vi "FestoCPX.Station.Laser.Shutterlock.vi"(8 "error in":errorcluster, 9 "Wait (T)":bool=TRUE, 10 "Shutterlock":bool) -> (0 "error out":errorcluster)   [LabVIEW 2015]
uses:
  FestoCPX.DO.Signal.ctl
  tools/EventLog/EventLog.EventSource.ctl
  tools/Translator/Translator.Message.ctl
  V7310/LowLevel/V7310.LaserStatus.ctl
  V7310/V7310.Data.Status.State.ctl
  FestoCPX.DO.Data.State.Set.vi
  V7310/LowLevel/V7310.Global.vi
  tools/EventLog/EventLog.CreateError(single).vi
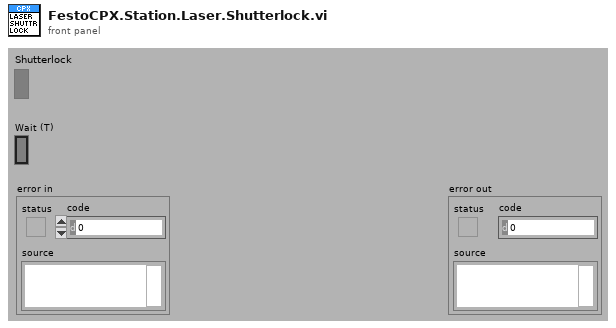
[diagram p1: front panel]
types:
  T1 = typedef "FestoCPX.DO.Signal.ctl" = enum16{"Safety Reset", "Air Main Valve", "Door Lock", "Button LED Start", "Button LED Stop", "Button LED Control", "Traffic LED Red", "Traffic LED Orange", "Traffic LED Green", "Horn", "Laser Interlock", "Laser Shutterlock", "Laser Fume Extractor", "Product Suction Gripper Slot 1 A", "Product Suction Gripper Slot 1 B", "Product Suction Gripper Slot 2 A", "Product Suction Gripper Slot 2 B", "Product Suction Gripper Slot 3 A", "Product Suction Gripper Slot 3 B", "Product Suction Gripper Slot 4 A", "Product Suction Gripper Slot 4 B", "Product Suction Gripper Final A", "Product Suction Gripper Final B", "Lamp", "Q1 Product Move Work", "Q1 Product Move Home", "Q2 Table Turn Work", "Q2 Table Turn Home", "Q3 Product Lift A", "Q3 Product Lift B", "Q4 Product Arm OK", "Q4 Product Arm NOK", "Q5 Product Arm Work"}
  T2 = typedef "Translator.Message.ctl" = enum16{"-", "Event confirmed", "Log out", "Log in", "Shutdown", "Cancel", "Start", "Begin time", "End time", "Duration", "Service Mode", "Ignore Results", "On", "Off", "OK", "NOK", "NOK %s", "Home", "Work", "Close", "Open", "In progress...", "Missing", "Empty", "Hardware failure", "Initial", "Error %d >> %s", "Error %d >> %s >> %s", "Msg %d >> %s", "Laser cmd error %s %d", "Laser cmd failed %s", "Laser cmd warning %s", "Laser disconnected", "Laser status %s", "Laser already started", "Laser job unkonwn %s", "Laser job missing %s", "Laser job select failure %s", "Laser marking timeout", "Laser marking aborted", "Unable to reset Laser Interlock (%s)", "Unable to trigger Laser. Laser not ready (%s)", "Starting %s", "Quitting %s", "Configured", "Initializing", "Quitting", "Loading", "Running", "Stopped", "Summary", "Laser", "Do you want to continue?", "Press confirm button", "Station is not based. Do you want to exit?", "Station requires changeover. Do you want to run the test?", "Test options are not set as default. Do you want to continue?", "Product not detected. Do you want to continue?", "Product scan failed. Do you want to continue?", "Calibration", "Log out?", "System", "All", "IDLE", "Translating...%s", "Not found", "Alarm %s", "Run", "Skip", "Abort", "Repeat", "Please wait...", "Database disconnected", "Database disconnected - changeover disabled!", "Login to database successful", "Login to database failed: %d; %s", "Unable to check the product status of reference %d - database disconnected", "Unable to set the product status of reference %d - database disconnected", "Variant file backup %s", "Read steps (%s)", "Result", "Station armed!", "Station requires changeover!", "Select reference number...", "EMERGENCY BUTTON - press Control button", "EMERGENCY DOOR - press Control button", "Resetting Emergency...", "Unable to reset safety circuit - Emergency Button pressed", "Unable to reset safety circuit - Emergency Side Door open", "Station not based", "Station based", "Station not empty", "Station basing...", "No order", "Press Start to begin new order", "Scanning new order", "Order NOK. Correct or scan again", "Order OK. Press Accept", "Order ready", "Revolver incorrect", "Revolver missing", "Revolver empty", "Container missing", "Offline results", "Door open", "Close the front door", "Press start button", "Done. Open the front door", "Error. Press Confirm button", "Remove product", "Confirm failure", "Running...", "Running...%.1f %%", "Pause", "Pause. NOK container missing", "Pause. OK container missing", "Pause. Revolver empty", "Pause. Revolver missing", "Pause.Revolver incorrect", "Stopping...", "Finalizing...", "Sequence folder '%s' is missing", "File '%s' is missing", "File '%s' is broken", "File '%s' is running", "Log file started (%s)", "Log file ended (%s)", "Log file ignored (%s)", "Log file exported (%s)", "Log file export failed (%s)", "Wrong serial number in log file", "Wrong reference number in log file", "Test steps are missing", "%s = %.3f", "Process param '%s' not found in DB", "Process param '%s' wrong order", "Process param '%s' value %.3f out of limits (%.3f; %.3f)", "Step%d param '%s' not found in DB", "Step%d param '%s' wrong order", "Step%d param '%s' value %.3f out of limits (%.3f; %.3f)", "Step%d EV '%s' not found in DB", "Step%d EV '%s' wrong order", "\"%s\" not found in DB", "\"%s\" wrong order", "\"%s\" value %.3f out of limits (%.3f; %.3f)", "\"%s\" not found in software", "Process initialized (%d)", "Process started", "Process done", "Process aborted", "Process aborted at work", "Process aborted at home", "Process error", "Process error at home", "Process error at work", "Product %s %d OK", "Product %s %d NOK", "Unable to unload the slot %s. Product missing in the slot", "Unable to unload the slot %s. Product already in the arm", "Unable to accept the product as OK. Product missing in slot %s", "Unable to accept the product as OK. Product could not drop into the container at slot %s", "Unable to accept the product as NOK. Product could not drop into the container at slot %s", "Scan failed. Error %s", "Scan failed. Scanner disconnected", "Scan failed. Wrong Wabco number %d, limit (%d,%d)", "Scan failed. Wrong serial number %d, limit (%d,%d)", "Scan failed. Wrong date %d, limit (%d,%d)", "Scan failed. Wrong product wabco number %d (expected %d)", "Scan failed. Wrong product serial number %d (expected > 0)", "Scan OK %s", "Scan failed. Unable to determine table position (%s)", "Scan failed. Timeout", "%s = %d", "%s = %d->%d", "Unable to set %s = %.2f - Air Pressure Inside off", "Unable to set digital output '%s' = %d", "Unable to activate air pressure inside - timeout", "Unable to activate air pressure inside - aborted", "Unable to switch on Air Main Valve - Air Pressure Inlet off", "Unable to switch on Air Main Valve - Door open", "Unable to switch off Air Main Valve - timeout", "Unable to switch off Air Main Valve - aborted", "Unable to rotate Table - timeout", "Unable to rotate Table - aborted", "Unable to rotate Table - Product Move not in Home position", "Unable to rotate Table - Air Pressure Inside off", "Unable to rotate Table - Product Lift A not in Home position", "Unable to rotate Table - Product Lift B not in Home position", "Unable to rotate Table - unlock before movement timeout", "Unable to rotate Table - lock after movement timeout", "Unable to move Table Lock to %s position - timeout", "Unable to move Table Lock to %s position - aborted", "Unable to move Table Lock to %s position - Air Pressure Inside off", "Unable to move Table Lock to %s position - Table not in position", "Unable to move Product Lift A to %s position - timeout", "Unable to move Product Lift B to %s position - timeout", "Unable to move Product Lift A to %s position - aborted", "Unable to move Product Lift B to %s position - aborted", "Unable to move Product Lift A to %s position - Air Pressure Inside off", "Unable to move Product Lift B to %s position - Air Pressure Inside off", "Unable to move Product Lift A to %s position - Table not locked", "Unable to move Product Lift B to %s position - Table not locked", "Unable to move Product Lift A to %s position - Product Arm not in Work position", "Unable to move Product Lift B to %s position - Product Arm not in Work position", "Unable to set Product Suction Gripper %s to %s - timeout", "Unable to set Product Suction Gripper %s to %s - aborted", "Unable to set Product Suction Gripper %s to %s - Air Pressure Inside off", "Unable to set Product Suction Gripper %s to %s - Table slot unkown", "Unable to move Product Arm to %s position - timeout", "Unable to move Product Arm to %s position - aborted", "Unable to move Product Arm to %s position - Air Pressure Inside off", "Unable to move Product Arm to %s position - Product Lift A not in Home position", "Unable to move Product Arm to %s position - Product Lift B not in Home position", "Unable to move Product to %s position - timeout", "Unable to move Product to %s position - aborted", "Unable to move Product to %s position - Air Pressure Inside off", "Unable to move Product to %s position - Table not in position"}
  T3 = typedef "EventLog.EventSource.ctl" = enum16{"All", "Gui", "Ref", "File", "Seq", "CPX", "Proda", "Laser", "Scan.P", "Scan.O"}
  T4 = typedef "V7310.Data.Status.State.ctl" = enum16{"Init", "Msg", "Error", "Abort", "Idle", "Run"}
  T5 = typedef "V7310.LaserStatus.ctl" = enum16{"-", "Initialize", "KeySwitchOpen", "TimeoutInterlock", "InterlockOpen", "StartUp", "ShutterlockOpen", "Standby", "Ready", "PrepareForMarking", "WaitForTrigger", "Marking"}
  T6 = typedef "V7310.Data.Status.ctl" = cluster{"State":T4, "LaserStatus":T5, "LaserStatusRaw":string, "Ref":refnum<k5>, "RTC TS":timestamp, "Conn TS":timestamp, "Msg":T7[], "JobInUse":string, "Jobs":string[], "Vars":T8[]}
  T7 = typedef "V7310.Message.Data.ctl" = cluster{"ID":i32, "Message":string}
  T8 = typedef "V7310.Job.Variable.ctl" = cluster{"Name":string, "Value":string}
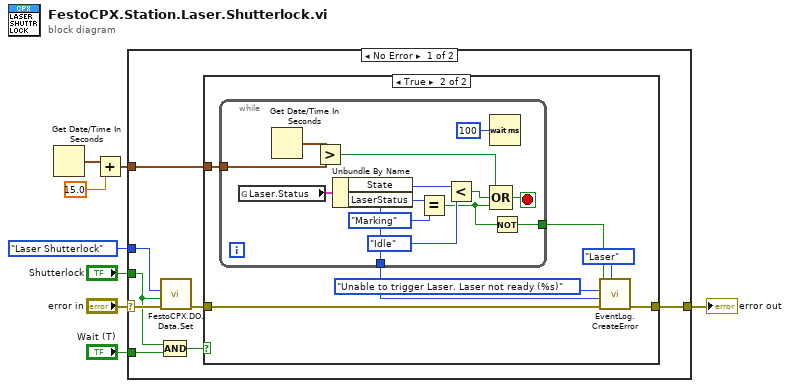
[diagram p0: block diagram]
diagram:
  n1 = Get Date/Time In Seconds() -> (seconds since 1Jan1904=w3:timestamp)
  n2 = Add(x=w3, y=15.0 ("x")) -> (x+y=w2:timestamp)
  n3 = case shown="No Error" "error in" {
    selector: "error in" -> [w16 w38]
    tunnel: [w13 w38] -> w8
    tunnel: "Shutterlock" -> [w11 _]
    tunnel: FestoCPX.DO.Signal."Laser Shutterlock" ("CPX.DO") -> [w15 _]
    tunnel: "Wait (T)" -> [w10 _]
    tunnel: w2 -> [w12 _]
    frame No Error {
      n4 = call-poly "FestoCPX.DO.Data.Set.vi"("error in (no error)"=w16, "State"=w11, "CPX.DO"=w15) -> ("error out"=w14:errorcluster)  [unwired: 8 in]
      n5 = Compound Arithmetic op=AND(w11, w10) -> (w9:bool)
      n6 = case shown="True" w9 {
        tunnel: w14 -> [w17 w20]
        tunnel: [w17 w24] -> w13
        tunnel: w12 -> [_ w23]
        frame False {
        }
        frame True {
          n7 = while {
            tunnel: w23 -> [w32]
            tunnel: [w27] -> w22
            tunnel: [w25] -> w18
            stop <- w29 stop-if-true
            n8 = global read "V7310.Global.vi" "Laser.Status"() -> (w37:T6)
            n9 = Get Date/Time In Seconds() -> (seconds since 1Jan1904=w31:timestamp)
            n10 = Greater?(x=w31, y=w32) -> (0:w30:bool)
            n11 = Unbundle By Name(w37) -> ("State"=w35:T4, "LaserStatus"=w25:T5)
            n12 = Equal?(x=w25, y=V7310.LaserStatus."Marking") -> (x = y?=w28:bool)
            n13 = Less?(x=w35, y=V7310.Data.Status.State."Idle" ("State")) -> (x < y?=w33:bool)
            n14 = Wait (ms)(milliseconds to wait=u32 100) -> ()  [unwired: 1 out]
            n15 = Compound Arithmetic op=OR(w30, w33, w28) -> (w29:bool)
            n16 = Not(x=w28) -> (.not. x?=w27:bool)
          }
          n17 = call-poly "EventLog.CreateError.vi"("Source (All)"=EventLog.EventSource."Laser", "error in"=w20, "arg"=w18, "msg"=Translator.Message."Unable to trigger Laser. Laser not ready (%s)", "create (T)"=w22) -> ("error out"=w24:errorcluster)  [unwired: 6 in]
        }
      }
    }
    frame Error {
    }
  }
  "error out" <- w8
